vi "XIPIN_10G_Ethernet_MAC_15_0.vi"   [LabVIEW 2017]
doc: "The LogiCORE?IP 10G Ethernet MAC core is designed to the IEEE 802.3 standard specification to provide a full-duplex Ethernet Media Access Controller (MAC). The core supports LAN/WAN mode operation and it provides support for VLAN and JUMBO frames. It also provides optional network management features including statistics gathering and flow control. The core is designed to seamlessly connect to the XAUI, RXAUI and the 10G Ethernet PCS/PMA LogiCOREs.\n------------------------------------\n<b>Need License</b> : Yes\n<b>Interface</b> : AXI4 AXI4-Stream"
uses:
  <vilib>/rvi/XilinxIP/XIPIN_XNode/niFpgaXIPIN.xnode
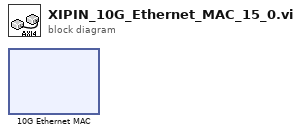
[diagram p0: block diagram]
diagram:
  n1 = xnode ("10G Ethernet MAC")() -> ()
